vi "CRC-16.vi"(11 "string":string) -> (2 "CRC-16":u16, 3 "string with CRC-16":string)   [LabVIEW 2015, in "PL Modbus Client.lvclass"]
doc: "Calculates CRC-16 and appends it to <B>string</B>."
uses:
  PL Modbus Client.lvclass
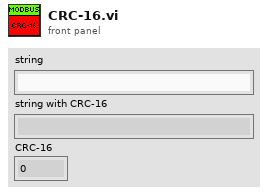
[diagram p1: front panel]
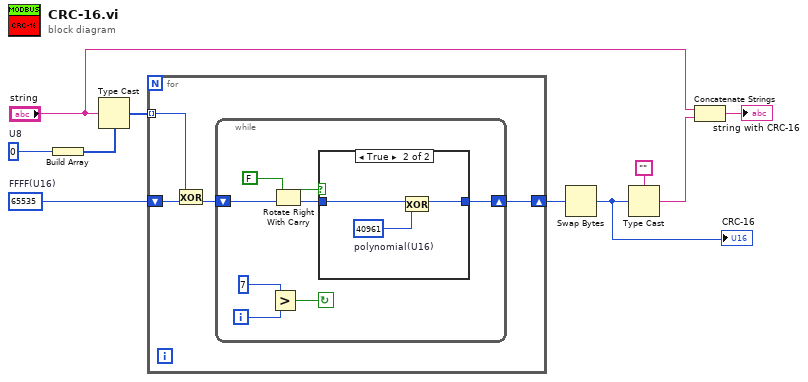
[diagram p0: block diagram]
diagram:
  w5 = u16 65535  # FFFF(U16)
  w10 = u8 0  # U8
  n1 = Build Array(w10) -> (w9:u8[])
  n2 = Type Cast(type=w9, x="string") -> (*(type *) &x=w8:u8[])
  n3 = for {
    tunnel: w8 -> [w14] mode=indexing
    shift-right: [w11] -> w4
    shift-left: w5 -> [w13]
    n4 = Exclusive Or(1:w13, 2:w14) -> (0:w12:u16)
    n5 = while {
      shift-right: [w18] -> w11
      shift-left: w12 -> [w16]
      i -> [w17]
      stop <- w15 continue-if-true
      n6 = Greater?(x=7, y=w17) -> (0:w15:bool)
      n7 = Rotate Right With Carry(2:w16, 3:FALSE) -> (0:w19:u16, 1:w20:bool)
      n8 = case shown="True" w20 {
        tunnel: w19 -> [w23 w26]
        tunnel: [w23 w24] -> w18
        frame False {
        }
        frame True {
          w25 = u16 40961  # polynomial(U16)
          n9 = Exclusive Or(1:w25, 2:w26) -> (0:w24:u16)
        }
      }
    }
  }
  n10 = Swap Bytes(anything=w4) -> (byte swapped=w3:u16)
  "CRC-16" <- w3
  n11 = Type Cast(type="", x=w3) -> (*(type *) &x=w6:string)
  n12 = Concatenate Strings("string", w6) -> (→"string with CRC-16":string)
